vi "Create Default Attributes.vi"(5 "Unique ID":string, 7 "Process Executive Ref":refnum<data-value>, 11 "Start Bug Remover in":refnum<class "Start Bug Remover.lvclass">) -> (3 "Start Bug Remover out":refnum<class "Start Bug Remover.lvclass">)   [LabVIEW 2019, in "Start Bug Remover.lvclass"]
uses:
  <vilib>/gpm_packages/@cs/Car-wash/Source/Process Steps/Start Bug Remover/Start Bug Remover.lvclass
  <vilib>/gpm_packages/@cs/test-executive/Source/Test Executive/ITestExecutive/ITest Executive.lvclass
  4839619c-72e2-48ab-b94d-b969cb54063f.vi
  <vilib>/Utility/error.llb/Error Cluster From Error Code.vi
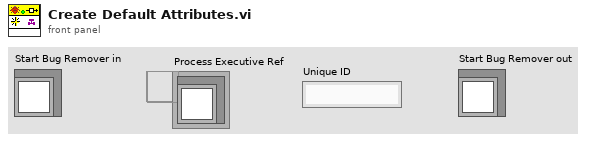
[diagram p1: front panel]
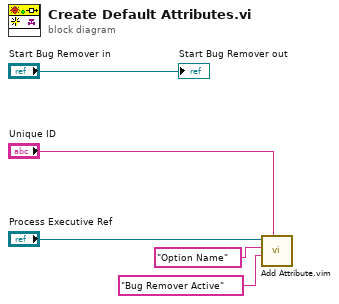
[diagram p0: block diagram]
diagram:
  n1 = call "Add Attribute.vim"("ID"="Unique ID", "Attribute"="Bug Remover Active" ("Item Name"), "Attribute Name"="Option Name" ("Item Name"), "Test Executive Ref"="Process Executive Ref") -> ()  [unwired: 4 in, 4 out]
  "Start Bug Remover out" <- "Start Bug Remover in"
